vi "Test_EndOfList_Wrap.vi"(8 "error in (no error)":errorcluster, 11 "TestCase in":refnum<class "TestStringList.lvclass">) -> (0 "error out":errorcluster, 3 "TestCase out":refnum<class "TestStringList.lvclass">)   [LabVIEW 2015, in "TestStringList.lvclass"]
uses:
  TestStringList.lvclass
  <vilib>/addons/_JKI Toolkits/VI Tester/TestCase.llb/TestCase.lvclass
  StringList.lvclass
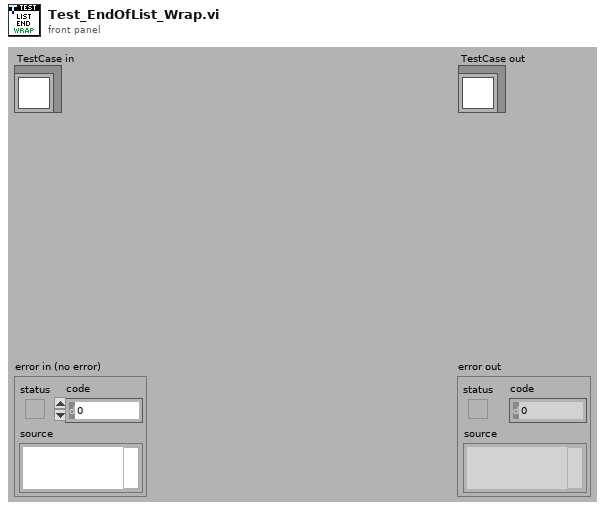
[diagram p1: front panel]
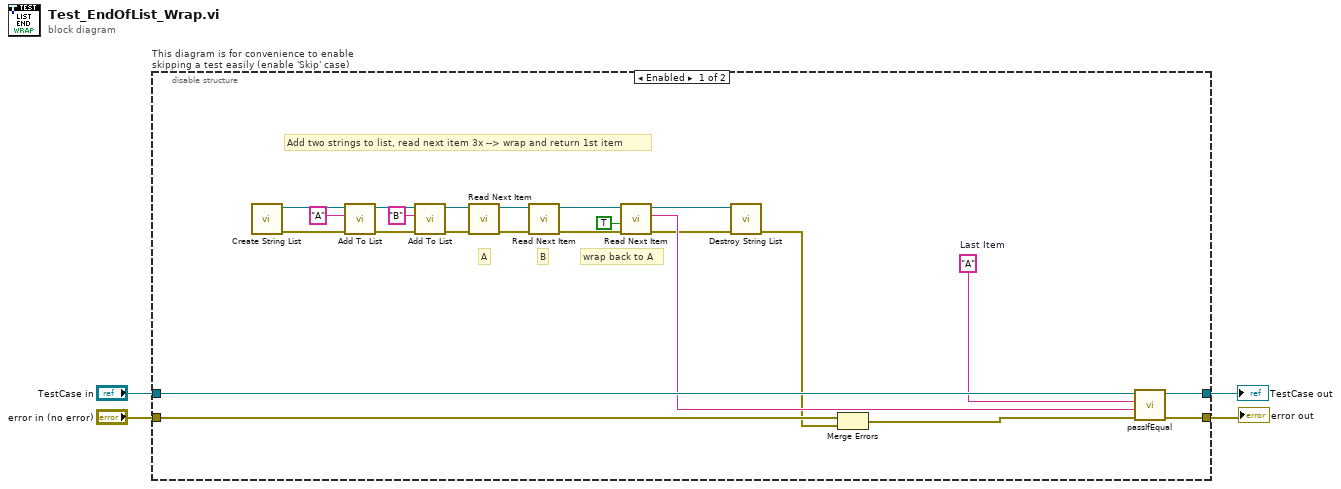
[diagram p0: block diagram]
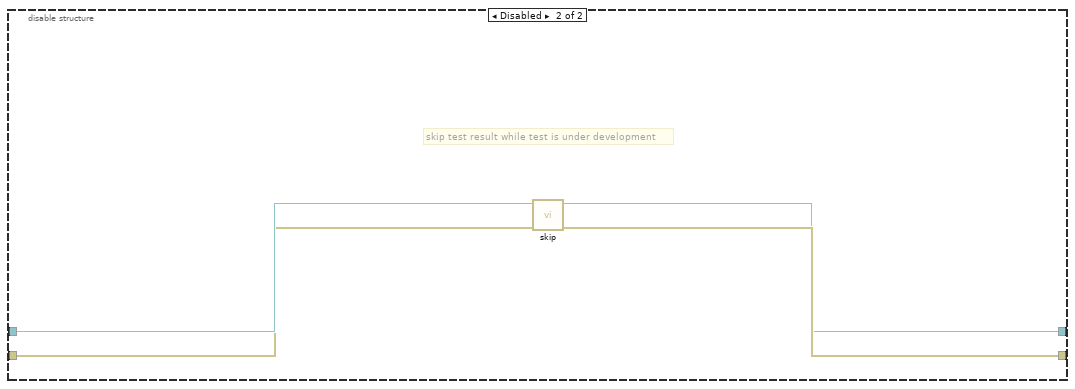
[diagram p2: hidden frame]
diagram:
  n1 = disable-structure "This diagram is for convenience to enable skipping a test easily (enable 'Skip' case)" shown="Enabled" {
    disable-tunnel: "TestCase in" -> [w27 w31]
    disable-tunnel: [w26 w29] -> w1
    disable-tunnel: [w25 w30] -> w3
    disable-tunnel: "error in (no error)" -> [w24 w28]
    frame Enabled {
      w23 = "A"  # Last Item
      # "wrap back to A"
      # "B"
      # "A"
      # "Add two strings to list, read next item 3x --> wrap and return 1st item"
      n2 = call "Create String List.vi"() -> ("error out"=w12:errorcluster, "StringList Reference"=w18:refnum<data-value>)  [unwired: 10 in]
      n3 = call "Add To List.vi"("error in (no error)"=w12, "Item"="A", "StringList Reference"=w18) -> ("error out"=w11:errorcluster, "StringList Reference"=w22:refnum<data-value>)  [unwired: 7 in]
      n4 = call "Add To List.vi"("error in (no error)"=w11, "Item"="B", "StringList Reference"=w22) -> ("error out"=w10:errorcluster, "StringList Reference"=w17:refnum<data-value>)  [unwired: 7 in]
      n5 = call "Read Next Item.vi"("error in (no error)"=w10, "StringList Reference"=w17) -> ("error out"=w9:errorcluster, "StringList Reference"=w20:refnum<data-value>)  [unwired: 6 in, 2 out]
      n6 = call "Read Next Item.vi"("error in (no error)"=w9, "StringList Reference"=w20) -> ("error out"=w8:errorcluster, "StringList Reference"=w15:refnum<data-value>)  [unwired: 6 in, 2 out]
      n7 = call "Read Next Item.vi"("error in (no error)"=w8, "Wrap? (F)"=TRUE, "StringList Reference"=w15) -> ("error out"=w7:errorcluster, "Item"=w19:string, "StringList Reference"=w13:refnum<data-value>)  [unwired: 5 in, 1 out]
      n8 = call "Destroy String List.vi"("error in (no error)"=w7, "StringList Reference"=w13) -> ("error out"=w5:errorcluster)  [unwired: 8 in, 1 out]
      n9 = Merge Errors(w24, w5) -> (w6:errorcluster)
      n10 = call-dynamic "passIfEqual.vi"("error in (no error)"=w6, "y"=w19, "x"=w23, "TestCase in"=w27) -> ("error out"=w25:errorcluster, "TestCase out"=w26:refnum<class "TestStringList.lvclass">)  [unwired: 6 in]
    }
    frame Disabled {
      # "skip test result while test is under development"
      n11 = call <vilib>:"skip.vi"("error in (no error)"=w28, "TestCase in"=w31) -> ("error out"=w30:errorcluster, "TestCase out"=w29:refnum<class "TestStringList.lvclass">)  [unwired: 8 in]
    }
  }
  "error out" <- w3
  "TestCase out" <- w1
